vi "Main Page VI Name.vi"(11 "CD Template in":refnum<class "NIVS_Inline HW Interface (Inline-Async).lvclass">) -> (2 "Main Page VI Name":string)   [LabVIEW 2020, in "NIVS_Inline HW Interface (Inline-Async).lvclass"]
uses:
  NIVS_Inline HW Interface (Inline-Async).lvclass
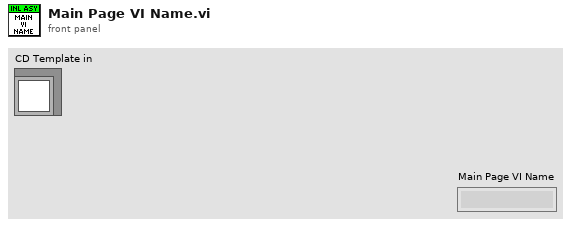
[diagram p1: front panel]
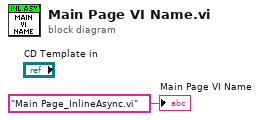
[diagram p0: block diagram]
diagram:
  "Main Page VI Name" <- "Main Page_InlineAsync.vi" ("Main Page VI Name")
